vi "Read Raw Data.vi"(8 "error in (no error)":errorcluster, 11 "Diode I-V in":refnum<class "Diode IV.lvclass">) -> (0 "error out":errorcluster, 2 "Raw Data":waveform(dbl), 3 "Diode I-V out":refnum<class "Diode IV.lvclass">)   [LabVIEW 2013, in "Diode Characterization.lvlib" / "Diode IV.lvclass"]
uses:
  Diode IV.lvclass
  Diode IV.lvclass/Diode IV.ctl
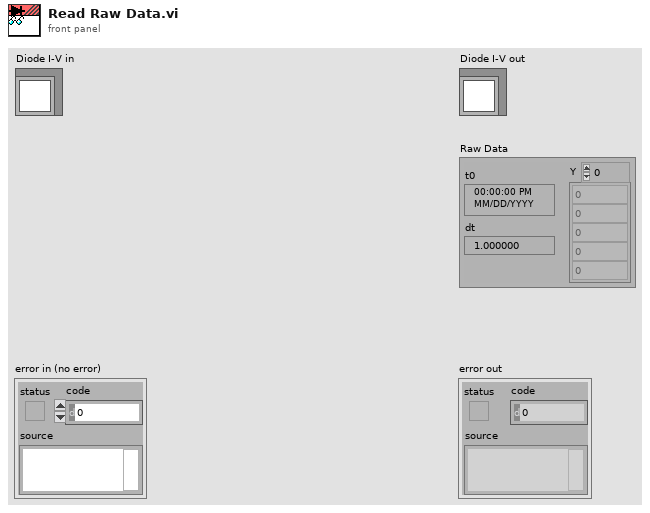
[diagram p1: front panel]
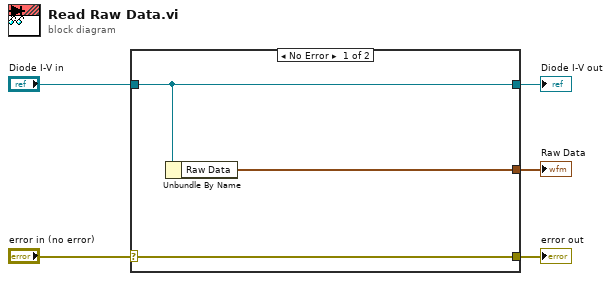
[diagram p0: block diagram]
diagram:
  n1 = case shown="No Error" "error in (no error)" {
    selector: "error in (no error)" -> [w8 w9]
    tunnel: [w8 w9] -> w4
    tunnel: [w7 w10] -> w2
    tunnel: "Diode I-V in" -> [w7 w10]
    tunnel: [w6 _] -> w1
    frame No Error {
      n2 = Unbundle By Name(w7) -> ("Raw Data"=w6:waveform(dbl))
    }
    frame Error {
    }
  }
  "error out" <- w4
  "Diode I-V out" <- w2
  "Raw Data" <- w1
